vi "GetPID.vi"() -> (0 "PID Gains":cluster{"P":dbl, "I":dbl, "D":dbl})   [LabVIEW 2014]
uses:
  <vilib>/Rock Robotics/Network Tables/SD Read Boolean.vi
  <vilib>/Rock Robotics/Network Tables/SD Read Number.vi
panel:
  in  "Gains Template":cluster{"P":dbl, "I":dbl, "D":dbl}
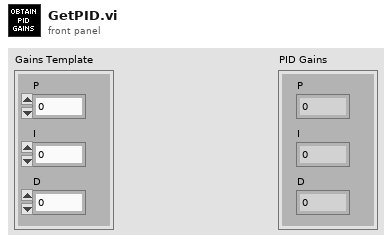
[diagram p1: front panel]
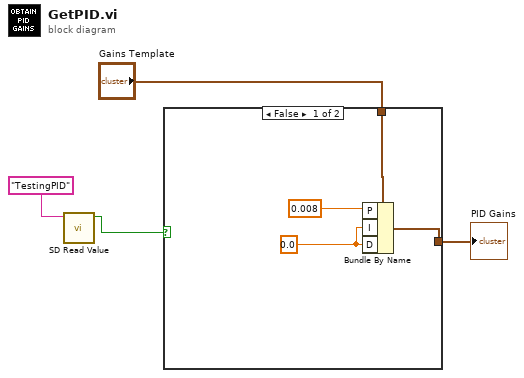
[diagram p0: block diagram]
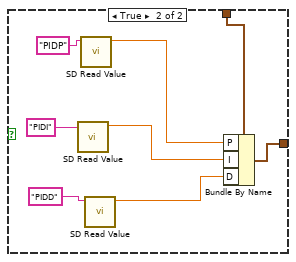
[diagram p2: hidden frame]
diagram:
  n1 = call-poly <vilib>:"SD Read Value.vi"("Name"="TestingPID") -> ("Boolean"=w3:bool)  [unwired: 8 in, 2 out]
  n2 = case shown="False" w3 {
    tunnel: [w8 w16] -> w2
    tunnel: "Gains Template" -> [w6 w15]
    frame False {
      w7 = 0.0
      n3 = Bundle By Name(cluster=w6, "P"=0.008, "I"=w7, "D"=w7) -> (w8:cluster{"P":dbl, "I":dbl, "D":dbl})
    }
    frame True {
      n4 = call-poly <vilib>:"SD Read Value.vi"("Name"="PIDI") -> ("Numeric"=w11:dbl)  [unwired: 8 in, 2 out]
      n5 = call-poly <vilib>:"SD Read Value.vi"("Name"="PIDP") -> ("Numeric"=w13:dbl)  [unwired: 8 in, 2 out]
      n6 = call-poly <vilib>:"SD Read Value.vi"("Name"="PIDD") -> ("Numeric"=w9:dbl)  [unwired: 8 in, 2 out]
      n7 = Bundle By Name(cluster=w15, "P"=w13, "I"=w11, "D"=w9) -> (w16:cluster{"P":dbl, "I":dbl, "D":dbl})
    }
  }
  "PID Gains" <- w2
